vi "Top Level State Machine.vi"(8 "error in":errorcluster, 9 "Buses":T2[](array[typedef])=[{"Devices"=[{"Number of Channels"=1, "Device Alias"="", "Icon Text"={"Line 1 text"="Bus", "Line 2 text"="Dev", "Line 3 text"="Ch", "Line 4 text"=""}}], "Pin Information"={"List of IO Names"=["sbRIO-9651 Socket\\PMOD1_Pin4_out", "sbRIO-9651 Socket\\PMOD1_Pin3_in", "sbRIO-9651 Socket\\PMOD1_Pin2_out", "sbRIO-9651 Socket\\PMOD1_Pin1_out"], "List of Enable Lines"=["sbRIO-9651 Socket\\PMOD1_Pin4_enable", "sbRIO-9651 Socket\\PMOD1_Pin3_enable", "sbRIO-9651 Socket\\PMOD1_Pin2_enable", "sbRIO-9651 Socket\\PMOD1_Pin1_enable"]}, "Replacement VI for DLU"=path "E:/Documents/Projects/SPIAPI/Pre-GitHub/Scripting Code 02_10_15 - Cleanup Time/Test/Replacement.vi", "Replacement VI for SPI Engine"=path ""}], 10 "Input Paths":T1={"Golden Template (Source) - (make relative)"=path "E:/Documents/Projects/SPIAPI/Github/SPIFramework/IONode", "Destination Generated Code (make relative)"=path "E:/Documents/Projects/SPIAPI/Github/SPIFramework/Test", "LabVIEW Project to Script"=path "E:/Documents/Projects/SPIAPI/Github/SPIFramework/Test/Test.lvproj", "Placement VI"=path "E:/Documents/Projects/SPIAPI/Github/SPIFramework/Test/TestVI.VI"}) -> (0 "error out":errorcluster)   [LabVIEW 2014, in "SPI Engine Scripting.lvlib"]
uses:
  SPI Engine Scripting.lvlib
  System.Windows.Forms
  State Machine/Controls/Bus Information.ctl
  State Machine/Controls/Device Information.ctl
  <vilib>/LabVIEW Icon API/API_Text.ctl
  State Machine/Controls/Pin Information.ctl
  State Machine/Controls/Input Paths.ctl
  Scripting States.ctl
  <vilib>/Utility/miscctls.llb/LVPointTypeDef.ctl
  <vilib>/LabVIEW Icon API/LabVIEW Icon API.lvlib
panel:
  out "Elapsed Time":dbl format="%<%H:%M:%S>t"
  in  "ProgressBar":refnum<k24>(container)
  out "Status":string
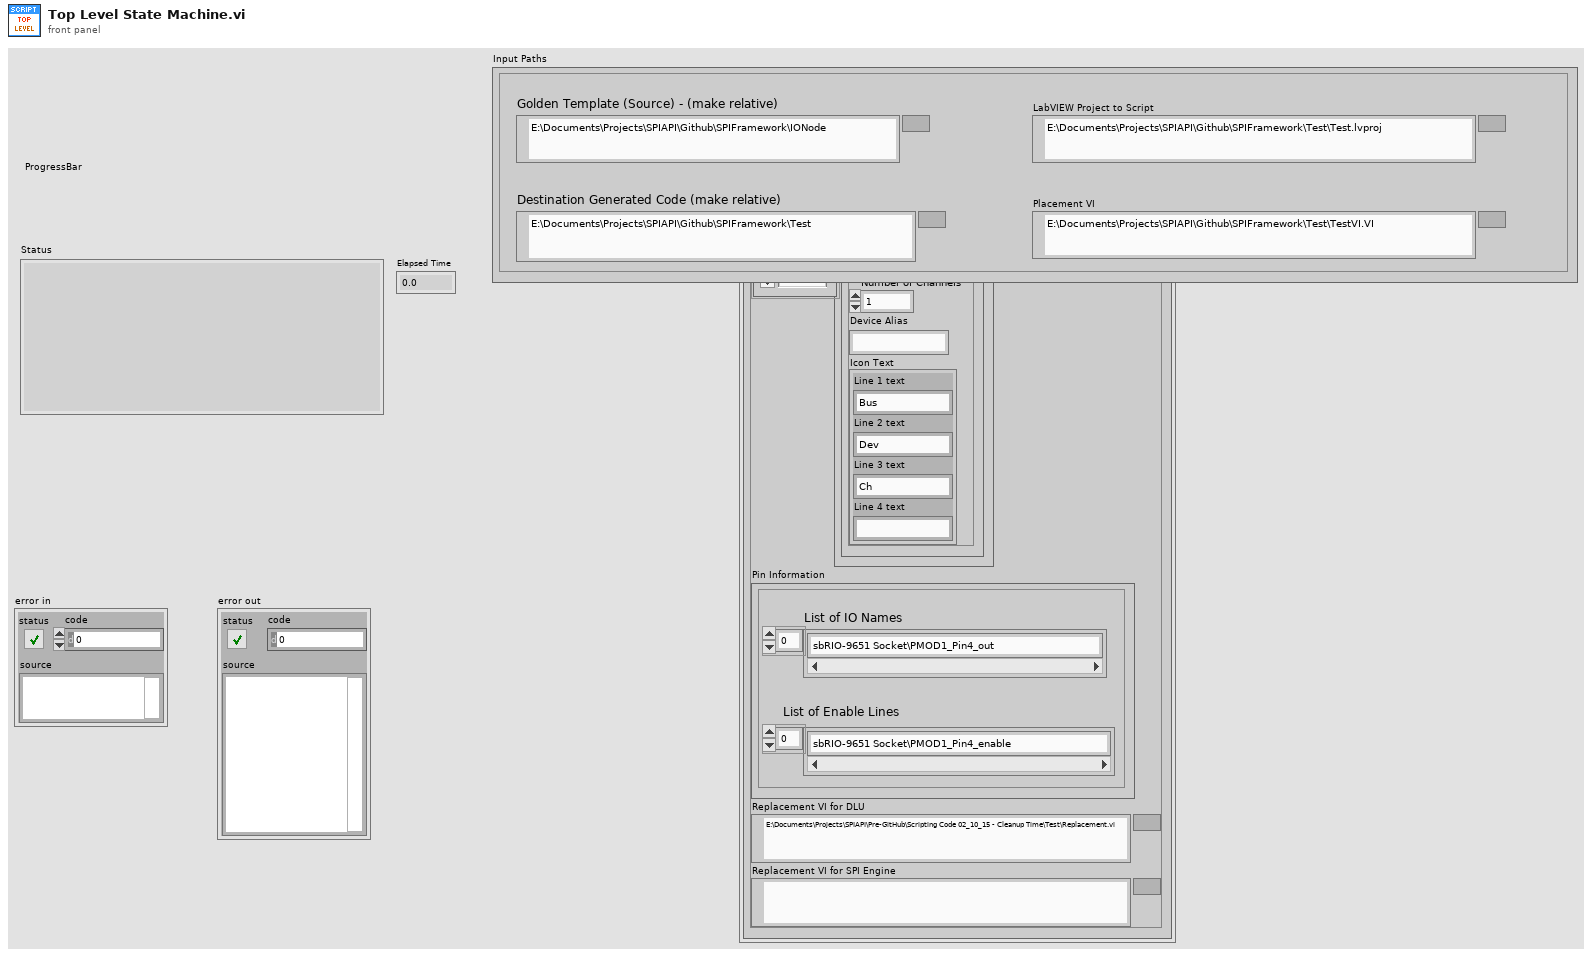
[diagram p1: front panel]
types:
  T1 = typedef "SPI Engine Scripting.lvlib/Input Paths.ctl" = cluster{"Golden Template (Source) - (make relative)":path, "Destination Generated Code (make relative)":path, "LabVIEW Project to Script":path, "Placement VI":path}
  T2 = typedef "SPI Engine Scripting.lvlib/Bus Information.ctl" = cluster{"Devices":T3[], "Pin Information":T5, "Replacement VI for DLU":path, "Replacement VI for SPI Engine":path}
  T3 = typedef "Device Information.ctl" = cluster{"Number of Channels":i32, "Device Alias":string, "Icon Text":T4}
  T4 = typedef "LabVIEW Icon API.lvlib/API_Text.ctl" = cluster{"Line 1 text":string, "Line 2 text":string, "Line 3 text":string, "Line 4 text":string}
  T5 = typedef "Pin Information.ctl" = cluster{"List of IO Names":string[], "List of Enable Lines":string[]}
  T6 = typedef "Initialization References.ctl" = cluster{"SPI Engine Virtual Folder":refnum<vi>, "ProgressBar out":refnum<k24>}
  T7 = typedef "Scripting States.ctl" = enum16{"Initialize", "Copy Template Bus Directory", "Modify Dequeue Commands", "Modify Enqueue Data", "Create FPGA VI", "Create Project FIFOs", "Create FPGA Data Nodes", "Place FPGA Data Nodes", "Update Node Count in Engine", "Expand FIFO Type Def", "Populate FIFO Names in Engine", "Modify I/O Pin Names", "Modify I/O Pin Enable", "Replace DLU", "Add Engine to Project", "Place SPI Engine", "Scripting Complete Check", "End"}
  T8 = enum32{"invalid VI type", "Standard VI", "Control VI", "Global VI", "Polymorphic VI", "Configuration VI", "SubSystem", "Facade VI", "Method VI", "Statechart Diagram VI"}
  T9 = typedef "LVPointTypeDef.ctl" = cluster{"Horizontal":i16, "Vertical":i16}
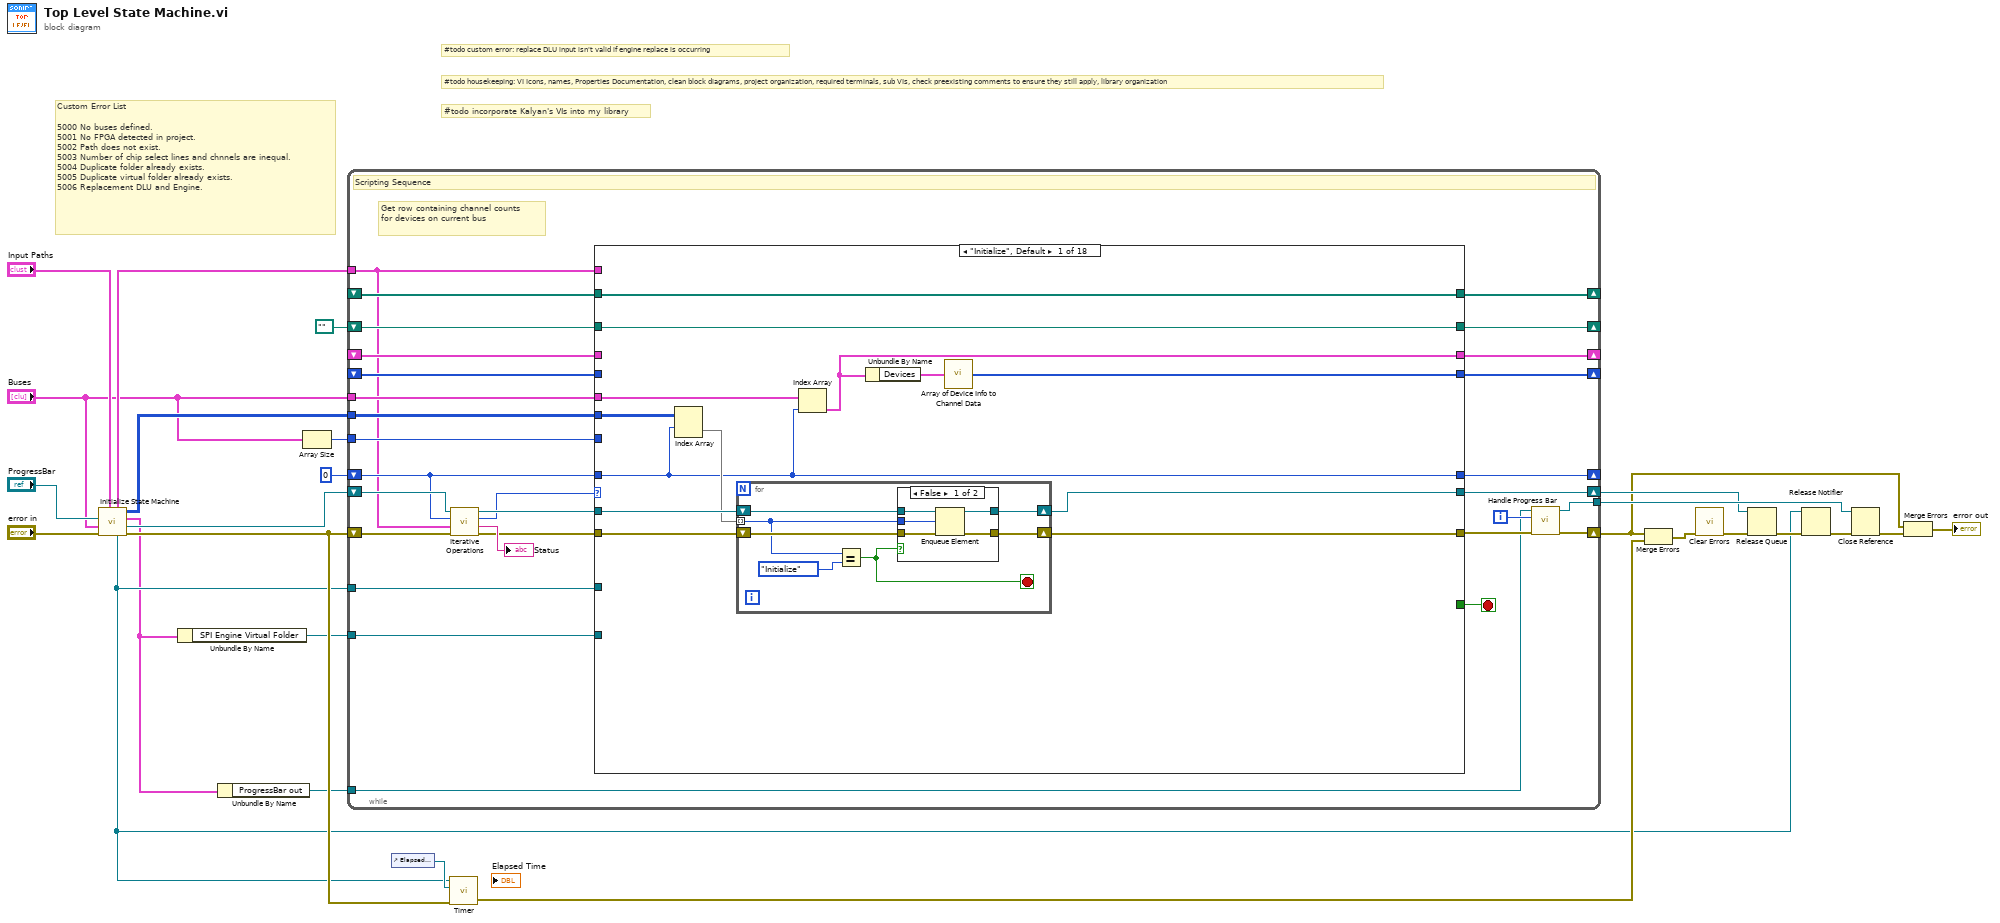
[diagram p0: block diagram]
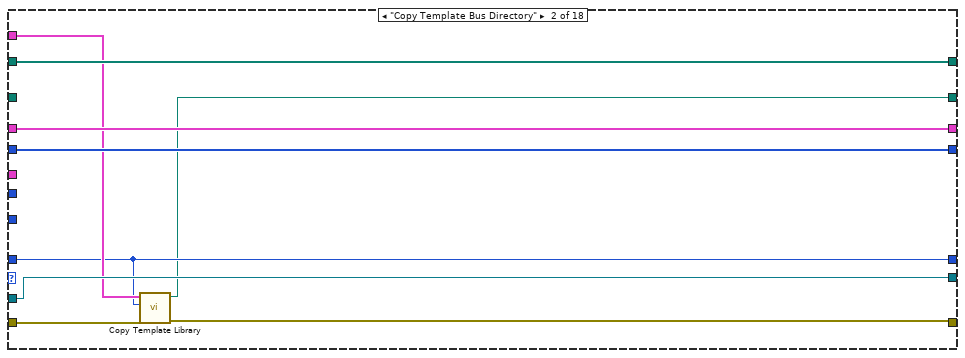
[diagram p3: hidden frame]
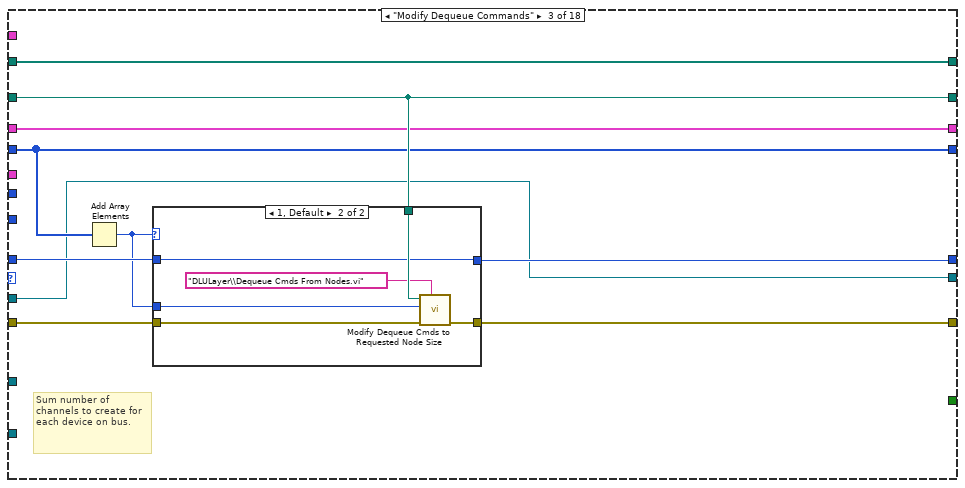
[diagram p4: hidden frame]
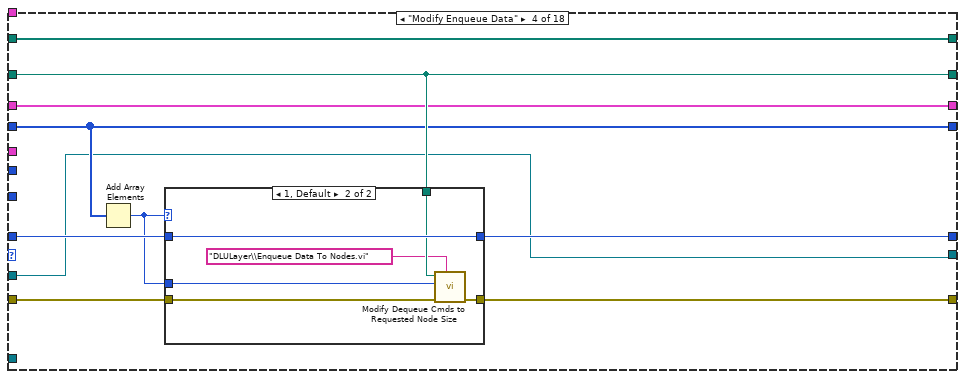
[diagram p6: hidden frame]
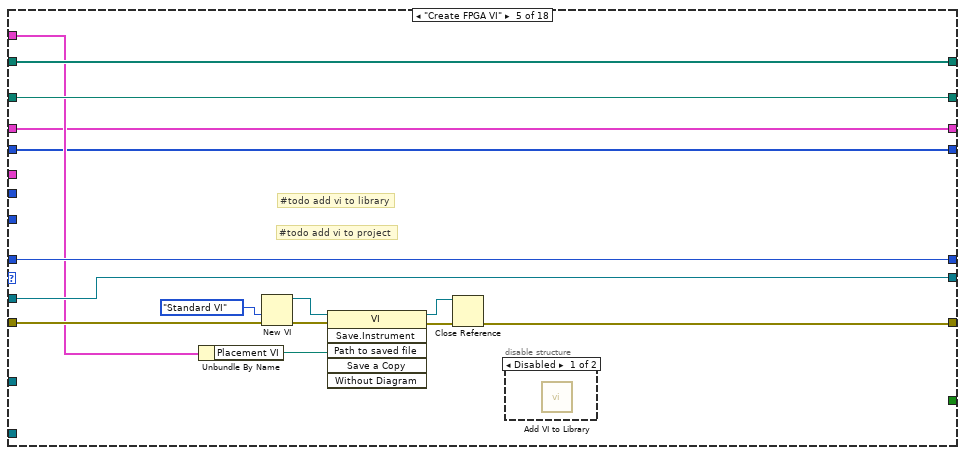
[diagram p8: hidden frame]
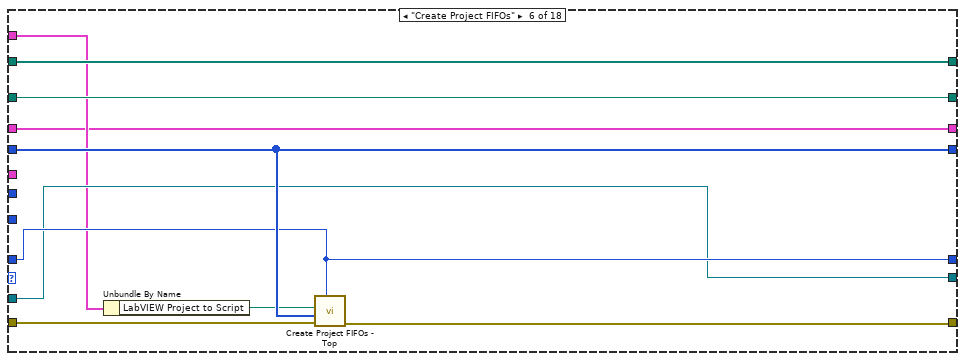
[diagram p10: hidden frame]
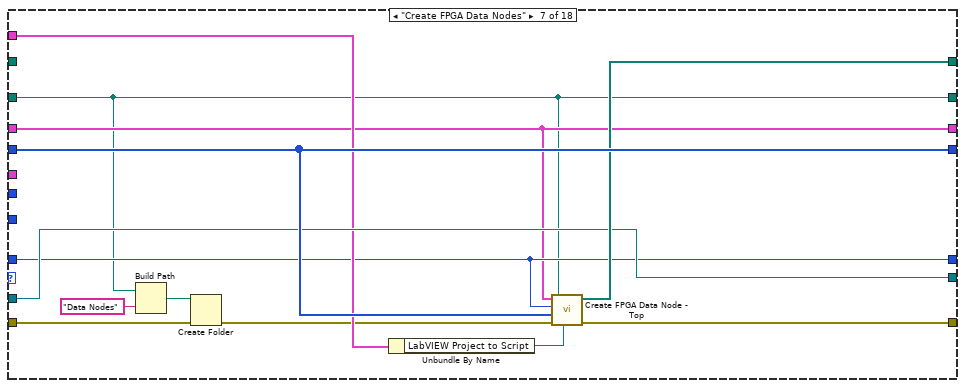
[diagram p11: hidden frame]
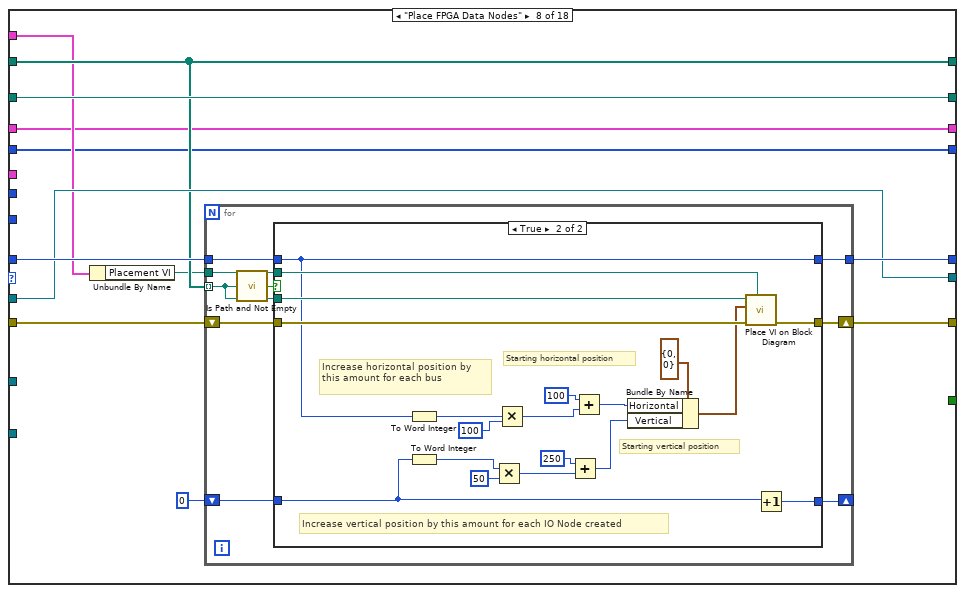
[diagram p12: hidden frame]
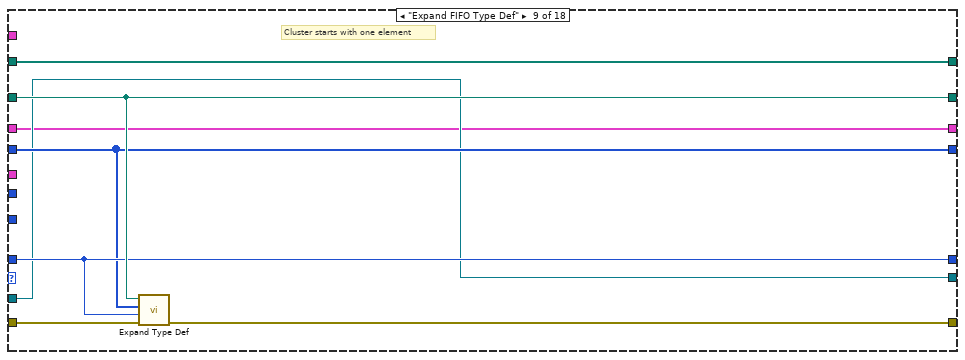
[diagram p14: hidden frame]
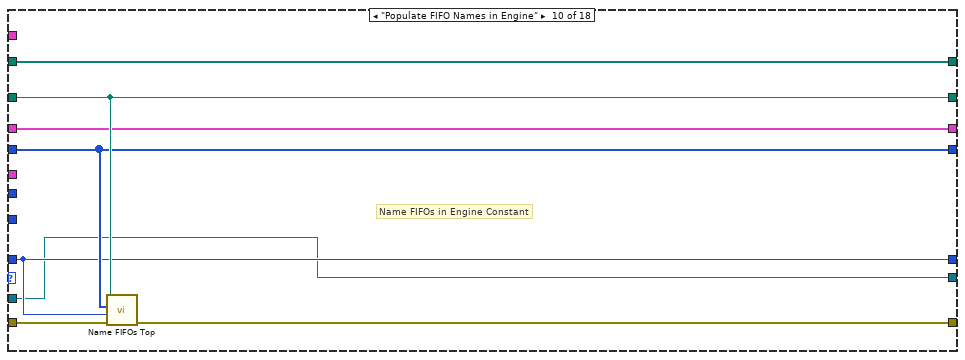
[diagram p15: hidden frame]
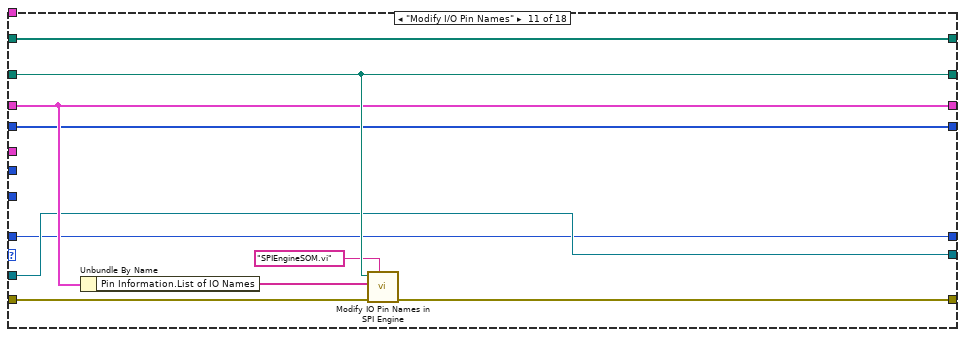
[diagram p16: hidden frame]
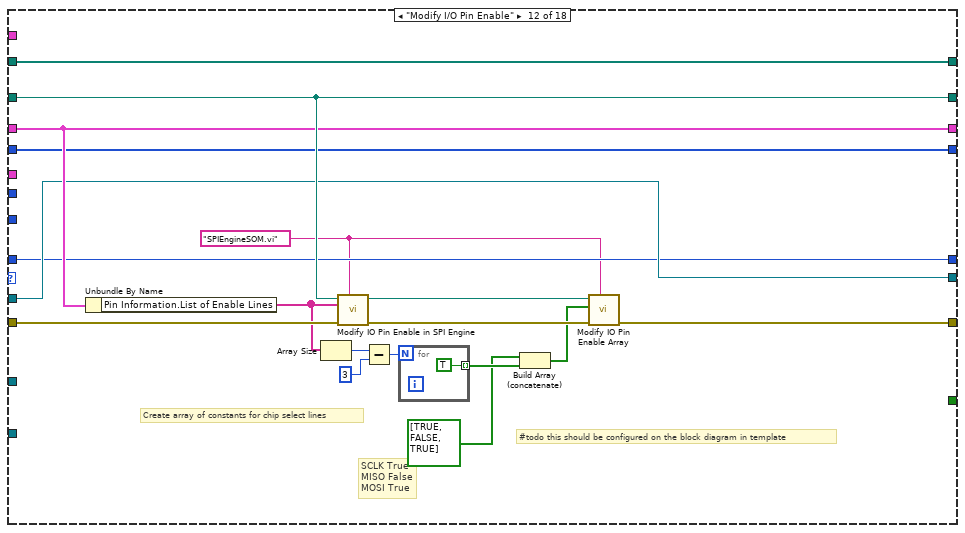
[diagram p17: hidden frame]
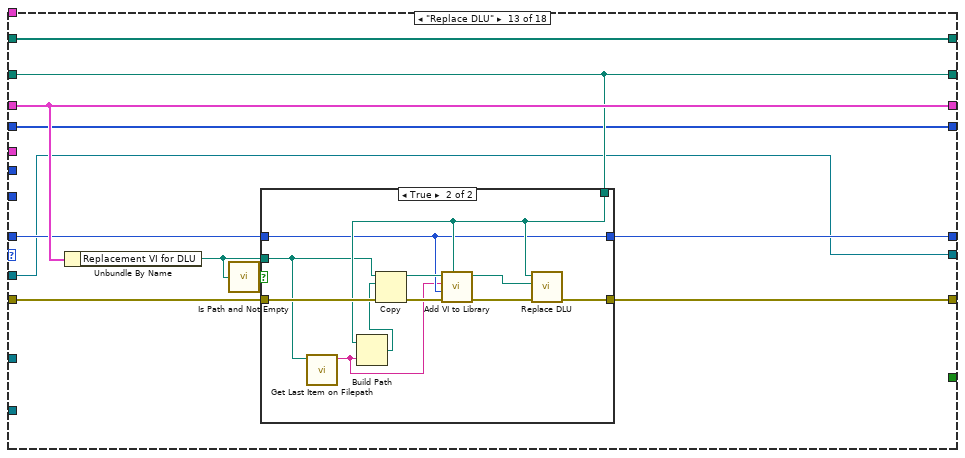
[diagram p18: hidden frame]
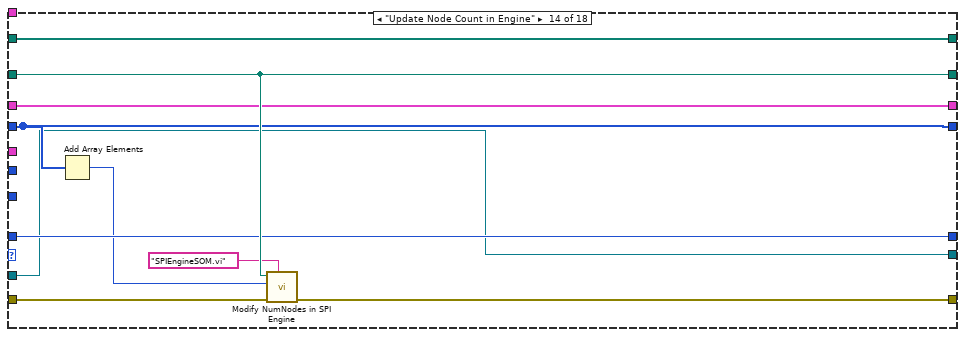
[diagram p20: hidden frame]
diagram:
  # "#todo custom error: replace DLU input isn't valid if engine replace is occurring"
  # "Custom Error List\n\n5000 No buses defined.\n5001 No FPGA detected in project.\n5002 Path does not exist.\n5003 Number of chip select lines and chnnels are inequal.\n5004 Duplicate folder already exists.\n5005 Duplicate virtual folder already exists.\n5006 Replacement DLU and Engine."
  # "#todo incorporate Kalyan's VIs into my library"
  # "#todo housekeeping: VI Icons, names, Properties Documentation, clean block diagrams, project organization, required terminals, sub VIs, check preexisting comments to ensure they still apply, library organization"
  n1 = call "Initialize State Machine.vi"("Input Paths (in)"="Input Paths", "error in"="error in", "Bus Info"="Buses", "ProgressBar in"="ProgressBar") -> ("error out"=w24:errorcluster, "State Queue"=w26:refnum<queue>, "References"=w2:T6, "State List"=w7:T7[][], "Notifier out"=w8:refnum<notifier>, "Inputs Paths (out)"=w6:T1)  [unwired: 2 in]
  n2 = Unbundle By Name(w2) -> ("SPI Engine Virtual Folder"=w1:refnum<vi>)
  n3 = Unbundle By Name(w2) -> ("ProgressBar out"=w3:refnum<k24>)
  n4 = Array Size(array="Buses") -> (size(s)=w4:i32)
  n5 = while {
    shift-right: [w47] -> w14
    shift-left: w24 -> [w43]
    shift-right: [w48] -> w19
    shift-left: w26 -> [w45]
    tunnel: [w54] -> w21
    tunnel: w3 -> [w52]
    shift-right: [w51] -> _
    shift-left: 0 ("Number of SPI Buses") -> [w44]
    shift-right: [w50] -> _
    shift-left: path "" ("Curent Bus Path") -> [w49]
    tunnel: w8 -> [w46]
    tunnel: "Buses" -> [w33]
    tunnel: w6 -> [w27]
    shift-right: [w38] -> _
    shift-left: _ -> [w37]
    tunnel: w7 -> [w35]
    tunnel: w4 -> [w34]
    shift-right: [w31] -> _
    shift-left: _ -> [w30]
    shift-right: [w32] -> _
    shift-left: _ -> [w29]
    tunnel: w1 -> [w28]
    i -> [w53]
    stop <- w36 stop-if-true
    # "Get row containing channel counts for devices on current bus"
    # "Scripting Sequence"
    n6 = call "Iterative Operations.vi"("error in"=w43, "Input Paths"=w27, "Current Bus Number"=w44, "Queue in"=w45) -> ("error out"=w39:errorcluster, "Current Status"=→"Status":string, "Next State"=w41:T7, "Queue out"=w42:refnum<queue>)  [unwired: 4 in]
    n7 = case shown="\"Initialize\", Default" w41 {
      tunnel: [w58 w83 w96 w113 w134 w147 w162 w172 w211 w219 w230 w239 w257 w281 w292 w313 w329 w343] -> w55
      tunnel: [w68 w91 w95 w114 w142 w148 w163 w174 w212 w220 w229 w240 w256 w280 w293 w315 w330 w348] -> w48
      tunnel: w39 -> [w57 w87 w100 w118 w139 w152 w157 w168 w216 w223 w234 w252 w263 w287 w297 w314 w331 w344]
      tunnel: w42 -> [w67 w91 w95 w114 w142 w148 w163 w174 w212 w220 w229 w240 w256 w280 w293 w315 w332 w348]
      tunnel: w49 -> [w56 _ w101 w119 w140 w150 w155 w176 w215 w224 w233 w250 w262 w286 w295 w312 w328 w350]
      tunnel: w29 -> [_ w89 w99 w117 w128 w151 w165 w169 w213 w222 w227 w237 w254 w283 w288 w308 w324 w339]
      tunnel: w44 -> [w59 w85 w98 w116 w133 w149 w160 w177 w214 w221 w226 w236 w259 w285 w294 w299 w338 w351]
      tunnel: [w59 w85 w97 w115 w133 w149 w160 w175 w214 w221 w226 w236 w258 w285 w294 w299 w336 w351] -> w51
      tunnel: [w56 w84 w101 w119 w140 w150 w155 w176 w215 w224 w233 w250 w262 w286 w295 w312 w328 w350] -> w50
      tunnel: w46 -> [_ _ _ _ _ _ _ _ _ _ _ _ _ _ _ _ _ w347]
      tunnel: w30 -> [_ w88 w93 w111 w129 w143 w158 w170 w209 w217 w232 w245 w264 w278 w298 w319 w325 w340]
      tunnel: w27 -> [_ w86 _ _ w131 w145 w161 w171 _ _ _ _ _ _ w290 w310 _ _]
      tunnel: [w64 w90 w94 w112 w132 w146 w164 w173 w210 w218 w228 w238 w255 w279 w291 w311 w327 w341] -> w38
      tunnel: w37 -> [w64 w90 w94 w112 w132 w146 _ w173 w210 w218 w228 w238 w255 w279 w291 w311 w327 w341]
      tunnel: [_ _ _ _ _ _ _ _ _ _ _ _ _ _ _ _ _ TRUE] -> w36
      tunnel: w35 -> [w66 _ _ _ _ _ _ _ _ _ _ _ _ _ _ _ _ _]
      tunnel: w34 -> [_ _ _ _ _ _ _ _ _ _ _ _ _ _ _ _ w326 _]
      tunnel: w33 -> [w62 _ _ _ _ _ _ _ _ _ _ _ _ _ _ _ _ _]
      tunnel: [w61 w89 w99 w117 w128 w151 w165 w169 w213 w222 w227 w237 w254 w283 w288 w308 w324 w339] -> w32
      tunnel: [w60 w88 w93 w111 w129 w143 w158 w170 w209 w217 w232 w245 w264 w278 w298 w319 w325 w340] -> w31
      tunnel: w28 -> [_ _ _ _ _ _ _ _ _ _ _ _ _ _ _ _ _ _]
      frame "Initialize", Default {
        n8 = Index Array(array=w66, index (row)=w59) -> (element=w65:T7[])  [unwired: 1 in]
        n9 = for {
          shift-right: [w75] -> w68
          shift-left: w67 -> [w74]
          shift-right: [w73] -> w58
          shift-left: w57 -> [w72]
          tunnel: w65 -> [w69] mode=indexing
          stop <- w70 stop-if-true
          n10 = Equal?(x=w69, y=Scripting_States."Initialize") -> (x = y?=w70:bool)
          n11 = case shown="False" w70 {
            tunnel: [w80 w82] -> w75
            tunnel: w74 -> [w79 w82]
            tunnel: [w78 w81] -> w73
            tunnel: w72 -> [w77 w81]
            tunnel: w69 -> [w76 _]
            frame False {
              n12 = Enqueue Element(queue=w79, element=w76, error in (no error)=w77) -> (queue out=w80:refnum<queue>, error out=w78:errorcluster)  [unwired: 1 in, 1 out]
            }
            frame True {
            }
          }
        }
        n13 = Index Array(array=w62, index=w59) -> (element=w60:T2)
        n14 = Unbundle By Name(w60) -> ("Devices"=w63:T3[])
        n15 = call "Array of Device Info to Channel Data.vi"("Array of Devices"=w63) -> ("Device Channels"=w61:i32[])
      }
      frame "Copy Template Bus Directory" {
        n16 = call "Copy Template Library.vi"("error in (no error)"=w87, "Current Bus Number"=w85, "Input Paths"=w86) -> ("error out"=w83:errorcluster, "Current Bus Path"=w84:path)  [unwired: 7 in]
      }
      frame "Modify Dequeue Commands" {
        # "Sum number of channels to create for each device on bus."
        n17 = Add Array Elements(numeric array=w99) -> (sum=w92:i32)
        n18 = case shown="1, Default" w92 {
          tunnel: [w103 w109] -> w96
          tunnel: w101 -> [_ w108]
          tunnel: w100 -> [w103 w107]
          tunnel: w92 -> [_ w104]
          tunnel: [w102 w105] -> w97
          tunnel: w98 -> [w102 w105]
          frame ..0 {
          }
          frame 1, Default {
            n19 = call "Modify Dequeue Cmds to Requested Node Size.vi"("VI to Code Relative Path"="DLULayer\\Dequeue Cmds From Nodes.vi", "Error In"=w107, "NumCases"=w104, "Source Root Path"=w108) -> ("Error Out"=w109:errorcluster)  [unwired: 5 in, 2 out]
          }
        }
      }
      frame "Modify Enqueue Data" {
        n20 = Add Array Elements(numeric array=w117) -> (sum=w110:i32)
        n21 = case shown="1, Default" w110 {
          tunnel: w119 -> [_ w124]
          tunnel: [w120 w125] -> w113
          tunnel: w118 -> [w120 w126]
          tunnel: w110 -> [_ w122]
          tunnel: [w121 w127] -> w115
          tunnel: w116 -> [w121 w127]
          frame ..0 {
          }
          frame 1, Default {
            n22 = call "Modify Dequeue Cmds to Requested Node Size.vi"("VI to Code Relative Path"="DLULayer\\Enqueue Data To Nodes.vi" ("VI to Code Rel Path"), "Error In"=w126, "NumCases"=w122, "Source Root Path"=w124) -> ("Error Out"=w125:errorcluster)  [unwired: 5 in, 2 out]
          }
        }
      }
      frame "Create FPGA VI" {
        # "#todo add vi to project"
        # "#todo add vi to library"
        n23 = Unbundle By Name(w131) -> ("Placement VI"=w130:path)
        n24 = New VI(8:w139, 9:T8."Standard VI" ("vi type (standard vi)")) -> (0:w138:errorcluster, 3:w137:refnum<vi>)  [unwired: 5 in]
        n25 = invoke class="VI" method="Save.Instrument"(reference=w137, error in=w138, "Path to saved file"=w130) -> (reference out=w135:refnum<vi>, error out=w136:errorcluster)  [unwired: 3 in, 4 out]
        n26 = Close Reference(reference=w135, error in (no error)=w136) -> (error out=w134:errorcluster)
        n27 = disable-structure shown="Disabled" {
          frame Disabled {
            n28 = call "Add VI to Library.vi"() -> ()  [unwired: 10 in, 2 out]
          }
          frame Enabled {
          }
        }
      }
      frame "Create Project FIFOs" {
        n29 = Unbundle By Name(w145) -> ("LabVIEW Project to Script"=w144:path)
        n30 = call "Create Project FIFOs - Top.vi"("Current Bus Number"=w149, "error in (no error)"=w152, "Device Channels"=w151, "LabVIEW Project to Script"=w144) -> ("error out"=w147:errorcluster)  [unwired: 7 in]
      }
      frame "Create FPGA Data Nodes" {
        n31 = Build Path(base path=w155, name or relative path="Data Nodes") -> (appended path=w153:path)
        n32 = Create Folder(path (use dialog)=w153, error in=w157) -> (error out=w156:errorcluster)  [unwired: 1 in, 2 out]
        n33 = Unbundle By Name(w161) -> ("LabVIEW Project to Script"=w159:path)
        n34 = call "Create FPGA Data Node - Top.vi"("LabVIEW Project to Script"=w159, "Curent Bus Path"=w155, "error in"=w156, "Device Channels"=w165, "Bus Number"=w160, "Device Info"=w158) -> ("error out"=w162:errorcluster, "New Node Paths"=w164:path[])  [unwired: 4 in]
      }
      frame "Place FPGA Data Nodes" {
        n35 = Unbundle By Name(w171) -> ("Placement VI"=w167:path)
        n36 = for {
          tunnel: w177 -> [w183]
          shift-right: [w181] -> w172
          shift-left: w168 -> [w186]
          tunnel: [w182] -> w175
          tunnel: w173 -> [w184] mode=indexing
          tunnel: w167 -> [w180]
          shift-right: [w178] -> _
          shift-left: i16 0 ("y") -> [w179]
          n37 = call <vilib>:"Is Path and Not Empty.vi"("path"=w184) -> ("Is Path and Not Empty?"=w185:bool)  [unwired: 4 in]
          n38 = case shown="True" w185 {
            tunnel: [w188 w207] -> w181
            tunnel: w186 -> [w188 w208]
            tunnel: w184 -> [_ w206]
            tunnel: [w189 w192] -> w182
            tunnel: w183 -> [w189 w192]
            tunnel: w180 -> [_ w205]
            tunnel: w179 -> [w187 w191]
            tunnel: [w187 w190] -> w178
            frame False {
            }
            frame True {
              # "Increase horizontal position by this amount for each bus"
              # "Starting horizontal position"
              # "Increase vertical position by this amount for each IO Node created"
              # "Starting vertical position"
              n39 = To Word Integer(number=w192) -> (16bit integer=w197:i16)
              n40 = To Word Integer(number=w191) -> (16bit integer=w199:i16)
              n41 = Multiply(x=w199, y=i16 50) -> (x*y=w202:i16)
              n42 = Multiply(x=w197, y=i16 100) -> (x*y=w195:i16)
              n43 = Add(x=i16 250, y=w202) -> (x+y=w204:i16)
              n44 = Add(x=i16 100, y=w195) -> (x+y=w194:i16)
              n45 = Bundle By Name(cluster=T9 {"Horizontal"=0, "Vertical"=0} ("location"), "Horizontal"=w194, "Vertical"=w204) -> (w193:T9)
              n46 = call "Place VI on Block Diagram.vi"("Path to Place VI"=w205, "error in"=w208, "Location to Place VI"=w193, "Path to VI Being Placed"=w206) -> ("error out"=w207:errorcluster)  [unwired: 7 in]
              n47 = Increment(x=w191) -> (x+1=w190:i16)
            }
          }
        }
      }
      frame "Expand FIFO Type Def" {
        # "Cluster starts with one element"
        n48 = call "Expand Type Def.vi"("error in (no error)"=w216, "Current Bus Number"=w214, "Device Channels"=w213, "Curent Bus Path"=w215) -> ("error out"=w211:errorcluster)  [unwired: 7 in]
      }
      frame "Populate FIFO Names in Engine" {
        # "Name FIFOs in Engine Constant"
        n49 = call "Name FIFOs Top.vi"("error in (no error)"=w223, "Current Bus Number"=w221, "Device Channels"=w222, "Curent Bus Path"=w224) -> ("error out"=w219:errorcluster)  [unwired: 7 in]
      }
      frame "Modify I/O Pin Names" {
        n50 = Unbundle By Name(w232) -> ("Pin Information.List of IO Names"=w231:string[])
        n51 = call "Modify IO Pin Names in SPI Engine.vi"("VI to Code Relative Path"="SPIEngineSOM.vi", "Error In"=w234, "List of IO Names"=w231, "Source Root Path"=w233) -> ("Error Out"=w230:errorcluster)  [unwired: 5 in, 2 out]
      }
      frame "Modify I/O Pin Enable" {
        w235 = "SPIEngineSOM.vi" ("VI to Code Relative Path")
        # "#todo this should be configured on the block diagram in template"
        # "Create array of constants for chip select lines"
        # "SCLK True\nMISO False\nMOSI True"
        n52 = Unbundle By Name(w245) -> ("Pin Information.List of Enable Lines"=w244:string[])
        n53 = Array Size(array=w244) -> (size(s)=w242:i32)
        n54 = call "Modify IO Pin Enable in SPI Engine.vi"("VI to Code Relative Path"=w235, "Error In"=w252, "List of Enable Lines"=w244, "Source Root Path"=w250) -> ("Error Out"=w251:errorcluster, "Source Root Path Out"=w249:path)  [unwired: 5 in, 1 out]
        n55 = Subtract(x=w242, y=3) -> (x-y=w243:i32)
        n56 = for {
          N: w243 -> [_]
          tunnel: [TRUE] -> w248 mode=indexing
        }
        n57 = Build Array (concatenate)(bool[] [TRUE, FALSE, TRUE], w248) -> (w246:bool[])
        n58 = call "Modify IO Pin Enable Array.vi"("VI to Code Relative Path"=w235, "Error In"=w251, "Enable"=w246, "Source Root Path"=w249) -> ("Error Out"=w239:errorcluster)  [unwired: 5 in, 2 out]
      }
      frame "Replace DLU" {
        n59 = Unbundle By Name(w264) -> ("Replacement VI for DLU"=w260:path)
        n60 = call <vilib>:"Is Path and Not Empty.vi"("path"=w260) -> ("Is Path and Not Empty?"=w261:bool)  [unwired: 4 in]
        n61 = case shown="True" w261 {
          tunnel: [w266 w277] -> w257
          tunnel: w263 -> [w266 w275]
          tunnel: w262 -> [_ w272]
          tunnel: w260 -> [_ w268]
          tunnel: w259 -> [w265 w270]
          tunnel: [w265 w270] -> w258
          frame False {
          }
          frame True {
            n62 = call "Get Last Item on Filepath.vi"("Replacement VI for SPI Engine"=w268) -> ("String"=w267:string)  [unwired: 10 in]
            n63 = Build Path(base path=w272, name or relative path=w267) -> (appended path=w271:path)
            n64 = Copy(8:w275, 10:w271, 11:w268) -> (0:w274:errorcluster, 3:w273:path)  [unwired: 2 in, 1 out]
            n65 = call "Add VI to Library.vi"("Current Bus Path"=w272, "error in"=w274, "Bus Number"=w270, "VI Name"=w267, "Path to new VI"=w273) -> ("error out"=w276:errorcluster, "Path to new IO Node"=w269:path)  [unwired: 5 in]
            n66 = call "Replace DLU.vi"("error in"=w276, "Replacement VI"=w269, "Current Bus Path"=w272) -> ("error out"=w277:errorcluster)  [unwired: 8 in]
          }
        }
      }
      frame "Update Node Count in Engine" {
        n67 = Add Array Elements(numeric array=w283) -> (sum=w282:i32)
        n68 = call "Modify NumNodes in SPI Engine.vi"("VI to Code Relative Path"="SPIEngineSOM.vi", "Error In"=w287, "Number of Nodes"=w282, "Source Root Path"=w286) -> ("Error Out"=w281:errorcluster)  [unwired: 4 in, 3 out]
      }
      frame "Add Engine to Project" {
        n69 = Unbundle By Name(w290) -> ("LabVIEW Project to Script"=w289:path)
        n70 = Unbundle By Name(w298) -> ("Replacement VI for SPI Engine"=w296:path)
        n71 = call "Add SPI Engine to Project and Lib.vi"("Number of SPI Buses in"=w294, "error in (no error)"=w297, "LabVIEW Project to Script"=w289, "Curent Bus Path"=w295, "Replacement VI for SPI Engine"=w296) -> ("error out"=w292:errorcluster)  [unwired: 6 in]
      }
      frame "Place SPI Engine" {
        # "Increase horizontal position by this amount for each bus"
        # "Starting horizontal position"
        n72 = Unbundle By Name(w319) -> ("Replacement VI for SPI Engine"=w317:path)
        n73 = To Word Integer(number=w299) -> (16bit integer=w303:i16)
        n74 = call <vilib>:"Is Path and Not Empty.vi"("path"=w317) -> ("Is Path and Not Empty?"=w316:bool)  [unwired: 4 in]
        n75 = case shown="False" w316 {
          tunnel: [w321 w323] -> w318
          tunnel: w317 -> [_ w323]
          tunnel: w312 -> [w320 _]
          frame False {
            n76 = Build Path(base path=w320, name or relative path="SPIEngineSOM.vi" ("VI to Code Relative Path")) -> (appended path=w321:path)
          }
          frame True {
          }
        }
        n77 = Multiply(x=w303, y=i16 100) -> (x*y=w305:i16)
        n78 = Add(x=i16 100, y=w305) -> (x+y=w302:i16)
        n79 = Bundle By Name(cluster=T9 {"Horizontal"=0, "Vertical"=0} ("location"), "Horizontal"=w302, "Vertical"=i16 150) -> (w300:T9)
        n80 = Unbundle By Name(w310) -> ("Placement VI"=w309:path)
        n81 = call "Place VI on Block Diagram.vi"("Path to Place VI"=w309, "error in"=w314, "Location to Place VI"=w300, "Path to VI Being Placed"=w318) -> ("error out"=w313:errorcluster)  [unwired: 7 in]
      }
      frame "Scripting Complete Check" {
        # "If yes, then all buses have been created, so end scripting. If not, then begin bus creation process."
        # "Is the current bus number equal to the total number of buses?"
        n82 = Increment(x=w338) -> (x+1=w336:i32)
        n83 = Equal?(x=w326, y=w336) -> (x = y?=w337:bool)
        n84 = Select(t=Scripting_States."End", s=w337, f=Scripting_States."Initialize") -> (s? t:f=w333:T7)
        n85 = Enqueue Element(queue=w332, element=w333, error in (no error)=w331) -> (queue out=w330:refnum<queue>, error out=w329:errorcluster)  [unwired: 1 in, 1 out]
      }
      frame "End" {
        (unwired) TRUE
        # "Stop Timer"
        n86 = call <vilib>:"Clear Errors.vi"("error in (no error)"=w344) -> ("error out"=w346:errorcluster)  [unwired: 5 in, 1 out]
        n87 = Send Notification(notification=TRUE, notifier=w347, error in (no error)=w346) -> (error out=w345:errorcluster)  [unwired: 1 out]
        n88 = Merge Errors(w344, w345) -> (w343:errorcluster)
      }
    }
    n89 = call "Handle Progress Bar.vi"("error in"=w55, "Numeric"=w53, ".NET Refnum in"=w52) -> ("error out"=w47:errorcluster, ".NET Refnum out"=w54:refnum<k24>)  [unwired: 7 in]
  }
  n90 = control-ref of="Elapsed Time"() -> (w16:refnum<vi>)
  n91 = call "Timer.vi"("error in (no error)"=w24, "DigNum Refnum"=w16, "Notifier in"=w8) -> ("error out"=w20:errorcluster)  [unwired: 8 in]
  n92 = Merge Errors(w14, w20) -> (w12:errorcluster)
  n93 = call <vilib>:"Clear Errors.vi"("error in (no error)"=w12) -> ("error out"=w13:errorcluster)  [unwired: 5 in, 1 out]
  n94 = Release Queue(queue=w19, error in (no error)=w13) -> (error out=w23:errorcluster)  [unwired: 1 in, 2 out]
  n95 = Release Notifier(notifier=w8, error in (no error)=w23) -> (error out=w22:errorcluster)  [unwired: 1 in, 2 out]
  n96 = Close Reference(reference=w21, error in (no error)=w22) -> (error out=w10:errorcluster)
  n97 = Merge Errors(w14, w10) -> (→"error out":errorcluster)
